vi "Create New Handled Error.vi"(1 "Error Number":i32, 2 "Reported Error":T3) -> (0 "Handled Error":T1)   [LabVIEW 2023, in "Error Manager.lvlib"]
doc: "Blank VI with error handling."
uses:
  Error Manager.lvlib
  Reported Error (cluster).ctl
  Public API VIs/Show Error Window Instruction (enum).ctl
  Handled Error (cluster).ctl
  Read-Unread Status (enum).ctl
panel:
  # "Input\nInputs to the VI"
  # "Development\nControls or indicators that are useful for development or testing, but which are not outputs of the VI."
  # "Output\nOutputs of the VI"
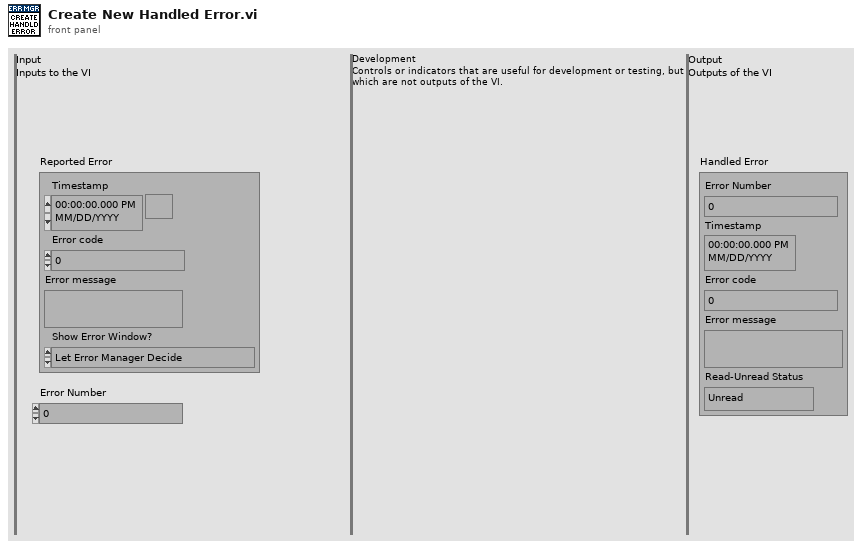
[diagram p1: front panel]
types:
  T1 = typedef "Error Manager.lvlib/Handled Error (cluster).ctl" = cluster{"Error Number":i32, "Timestamp":timestamp, "Error code":i32, "Error message":string, "Read-Unread Status":T2}
  T2 = typedef "Error Manager.lvlib/Read-Unread Status (enum).ctl" = enum16{"Unread", "Read"}
  T3 = typedef "Error Manager.lvlib/Reported Error (cluster).ctl" = cluster{"Timestamp":timestamp, "Error code":i32, "Error message":string, "Show Error Window?":T4}
  T4 = typedef "Error Manager.lvlib/Show Error Window Instruction (enum).ctl" = enum16{"Let Error Manager Decide", "Show", "Do Not Show"}
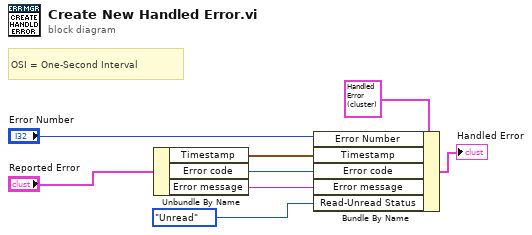
[diagram p0: block diagram]
diagram:
  # "OSI = One-Second Interval"
  n1 = Unbundle By Name("Reported Error") -> ("Timestamp"=w4:timestamp, "Error code"=w3:i32, "Error message"=w2:string)
  n2 = Bundle By Name(cluster=T1 {"Error Number"=0, "Timestamp"=timestamp(0 s since 1904-01-01), "Error code"=0, "Error message"="", "Read-Unread Status"=enum."Unread"} ("Handled Error"), "Error Number"="Error Number", "Timestamp"=w4, "Error code"=w3, "Error message"=w2, "Read-Unread Status"=Read-Unread_Status_(enum)."Unread") -> (→"Handled Error":T1)
